vi "Set Transform.vi"(8 "error in (no error)":errorcluster, 9 "Offset":cluster{"x":sgl, "y":sgl}, 10 "Matrix":T1=[[1.0, 0.0], [0.0, 1.0]], 11 "face":i64) -> (0 "error out":errorcluster, 3 "face 2":i64)   [LabVIEW 2023, in "Freetype Drawer.lvlib"]
uses:
  Freetype Drawer.lvlib
  <vilib>/Analysis/Matrix/Datatypes/RealMatrix.ctl
  libfreetype.dll
  <vilib>/Analysis/Matrix/NI_Matrix.lvlib
panel:
  out "32bit integer":cluster{"x":i32, "y":i32}
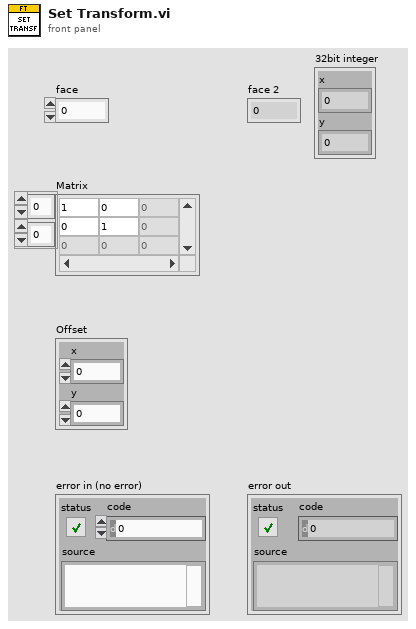
[diagram p1: front panel]
types:
  T1 = typedef "NI_Matrix.lvlib/RealMatrix.ctl" = dbl[][]
  T2 = cluster{"Matrix[0]":dbl, "Matrix[1]":dbl, "Matrix[2]":dbl, "Matrix[3]":dbl}
  T3 = cluster{"Matrix[0]":i32, "Matrix[1]":i32, "Matrix[2]":i32, "Matrix[3]":i32}
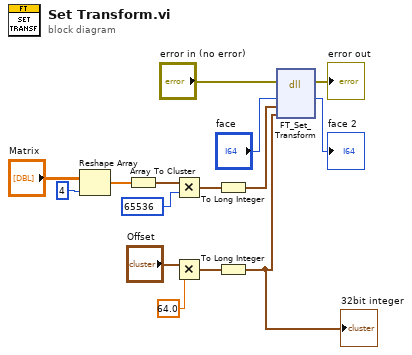
[diagram p0: block diagram]
diagram:
  n1 = Reshape Array("Matrix", 4 ("dimension size")) -> (w5:dbl[])
  n2 = Array To Cluster(array=w5) -> (cluster=w3:T2)
  n3 = Multiply(x=w3, y=65536) -> (x*y=w9:T2)
  n4 = Multiply(x="Offset", y=sgl 64.0) -> (x*y=w10:cluster{"x":sgl, "y":sgl})
  n5 = To Long Integer(number=w9) -> (32bit integer=w7:T3)
  n6 = To Long Integer(number=w10) -> (32bit integer=w2:cluster{"x":i32, "y":i32})
  "32bit integer" <- w2
  n7 = dll-call lib="E:/Labview/LV 2023/Libs/LV Symbol/Freetype Drawer/libfreetype.dll" fn="FT_Set_Transform"(error in="error in (no error)", "face"="face", "matrix"=w7, "delta"=w2) -> (error out=→"error out":errorcluster, "face"=→"face 2":i64)  [unwired: 5 in, 1 out]
